vi "joystick control MS.vi"() -> ()   [LabVIEW 2014]
uses:
  <vilib>/Utility/inputDevices.llb/joystickAcquire.vi
  <vilib>/Utility/inputDevices.llb/closeJoystick.vi
panel:
  out "V axis 8":i32
  out "V axis 7":i32
  out "V axis 6":i32
  out "V axis 5":i32
  out "V axis 4":i32
  out "V axis 3":i32
  out "V axis 2":i32
  out "V axis":i32
  out "U axis":i32
  in  "stop 2":bool
  in  "device index":i32
  out "joystick info":T1(array[cluster])
  out "Z axis":i32
  out "Y axis":i32
  out "X axis":i32
  out "error out":errorcluster
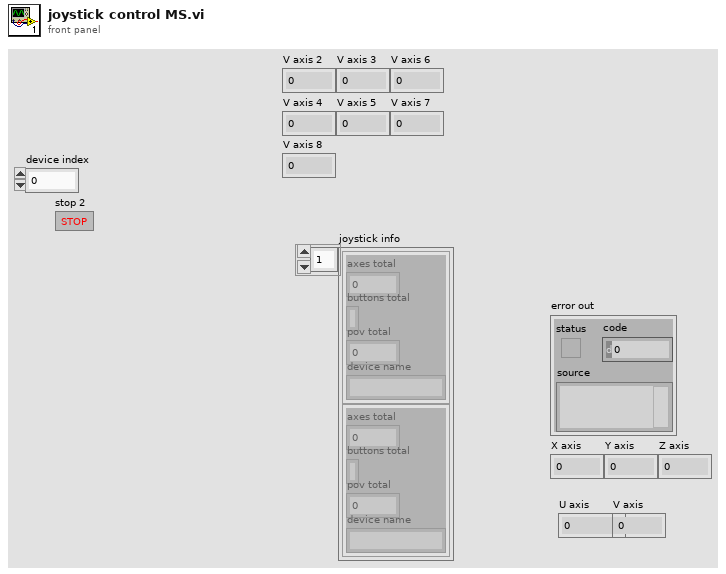
[diagram p1: front panel]
types:
  T1 = cluster{"axes total":u32, "buttons total":u32, "pov total":u32, "device name":string}[]
  T2 = cluster{"X axis":i32, "Y axis":i32, "Z axis":i32, "X axis rotation":i32, "Y axis rotation":i32, "Z axis rotation":i32, "U axis":i32, "V axis":i32}
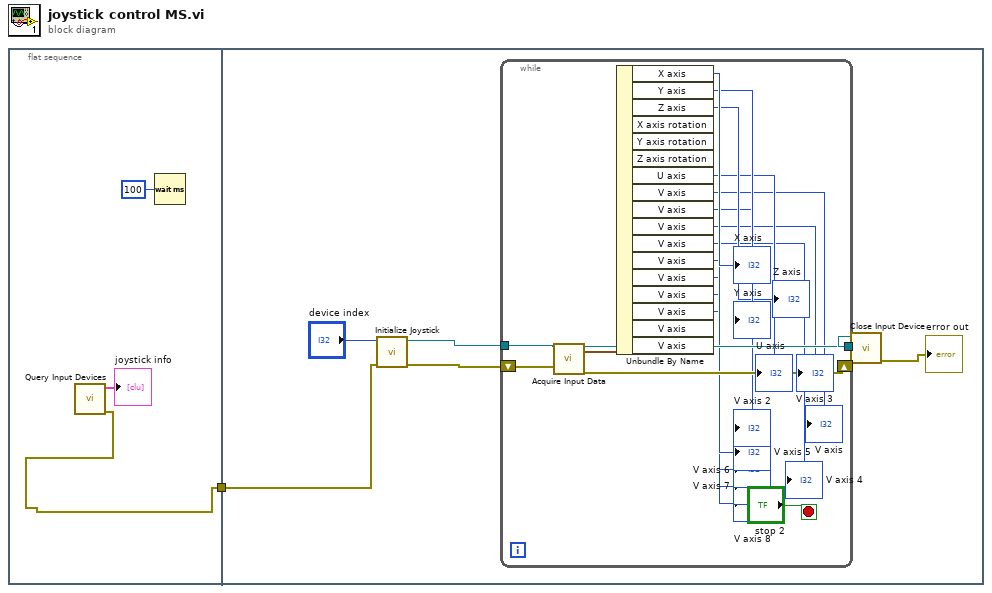
[diagram p0: block diagram]
diagram:
  n1 = flat-sequence {
    tunnel: [w3] -> w1
    tunnel: w1 -> [w5]
    frame #0 {
      n2 = call <vilib>:"Query Input Devices.vi"() -> ("error out"=w3:errorcluster, "joystick info"=→"joystick info":T1)  [unwired: 8 in, 2 out]
      n3 = Wait (ms)(milliseconds to wait=u32 100) -> ()  [unwired: 1 out]
    }
    frame #1 {
      n4 = call <vilib>:"Initialize Joystick.vi"("error in (no error)"=w5, "device index"="device index") -> ("error out"=w10:errorcluster, "device ID"=w9:refnum<k1>)  [unwired: 8 in]
      n5 = while {
        tunnel: w9 -> [w29]
        shift-right: [w22] -> w8
        shift-left: w10 -> [w27]
        tunnel: [w21] -> w6
        stop <- "stop 2" stop-if-true
        n6 = call-poly <vilib>:"Acquire Input Data.vi"("device ID"=w29, "error in (no error)"=w27) -> ("device ID 2"=w21:refnum<k1>, "axis info"=w28:T2, "error out"=w22:errorcluster)  [unwired: 13 in, 2 out]
        n7 = Unbundle By Name(w28) -> ("X axis"=→"X axis":i32, "Y axis"=→"Y axis":i32, "Z axis"=→"Z axis":i32, "U axis"=→"U axis":i32, "V axis"=→"V axis":i32, "V axis"=→"V axis 2":i32, "V axis"=→"V axis 3":i32, "V axis"=→"V axis 4":i32, "V axis"=→"V axis 5":i32, "V axis"=→"V axis 6":i32, "V axis"=→"V axis 7":i32, "V axis"=→"V axis 8":i32)  [unwired: 5 out]
      }
      n8 = call-poly <vilib>:"Close Input Device.vi"("error in (no error)"=w8, "device ID"=w6) -> ("error out"=→"error out":errorcluster)  [unwired: 8 in]
    }
  }
